vi "ReadCICDPathConfig.vi"(8 "error in (no error)":errorcluster, 11 "Workspace Path":path=path "E:/sw-deps-monitor") -> (0 "error out":errorcluster, 3 "CICD Path Config Out":T1)   [LabVIEW 2023, in "CheckModifiedVIs.lvlib"]
uses:
  CheckModifiedVIs/CheckModifiedVIs.lvlib
  Typedefs/CICDPathConfigs.ctl
  <vilib>/Utility/config.llb/NI_LVConfig.lvlib
  Reusables.lvlib
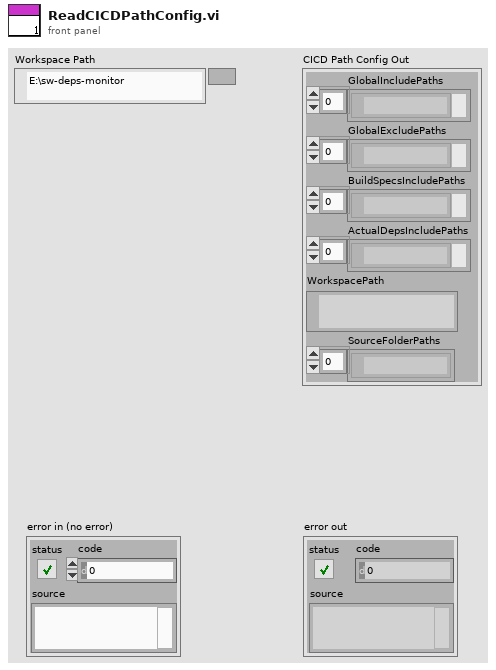
[diagram p1: front panel]
types:
  T1 = typedef "Reusables.lvlib/CICDPathConfigs.ctl" = cluster{"GlobalIncludePaths":path[], "GlobalExcludePaths":path[], "BuildSpecsIncludePaths":path[], "ActualDepsIncludePaths":path[], "WorkspacePath":path, "SourceFolderPaths":path[]}
  T2 = typedef "NI_LVConfig.lvlib/Config Data RefNum.ctl" = refnum<k1>
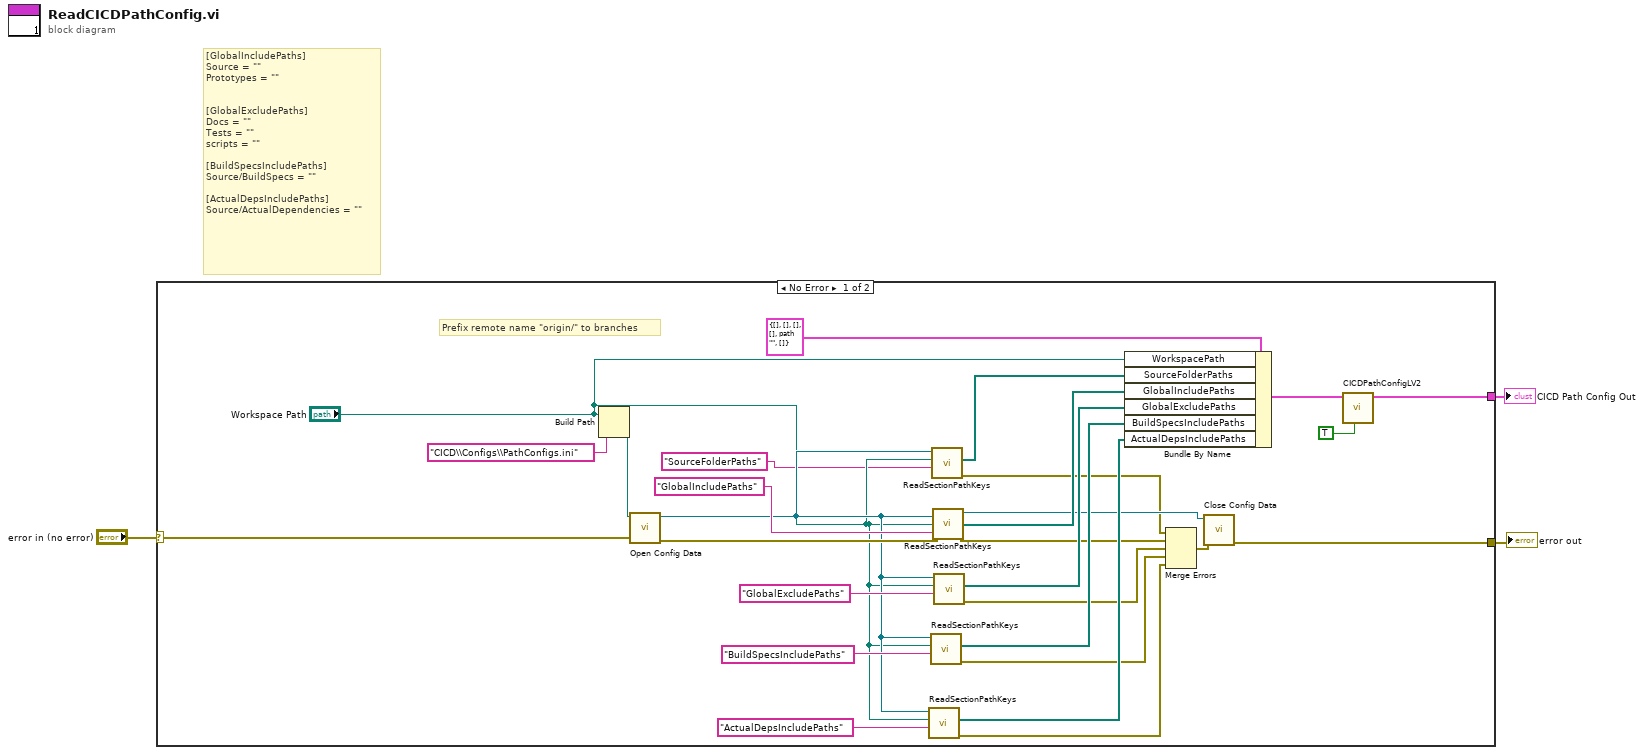
[diagram p0: block diagram]
diagram:
  # "[GlobalIncludePaths]\nSource = \"\"\nPrototypes = \"\"\n\n\n[GlobalExcludePaths]\nDocs = \"\"\nTests = \"\"\nscripts = \"\"\n\n[BuildSpecsIncludePaths]\nSource/BuildSpecs = \"\"\n\n[ActualDepsIncludePaths]\nSource/ActualDependencies = \"\""
  n1 = case shown="No Error" "error in (no error)" {
    selector: "error in (no error)" -> [w31 w32]
    tunnel: [w12 w32] -> w2
    tunnel: [w9 _] -> w1
    frame No Error {
      # "Prefix remote name \"origin/\" to branches"
      n2 = Build Path(base path="Workspace Path", name or relative path="CICD\\Configs\\PathConfigs.ini" ("CICD Path Config Rel")) -> (appended path=w30:path)
      n3 = call <vilib>:"Open Config Data.vi"("error in (no error)"=w31, "configuration file path"=w30) -> ("error out"=w28:errorcluster, "refnum"=w8:T2)  [unwired: 7 in, 1 out]
      n4 = call "ReadSectionPathKeys.vi"("section"="ActualDepsIncludePaths", "Workspace Path"="Workspace Path", "Refnum in"=w8) -> ("error out"=w15:errorcluster, "Paths"=w19:path[])  [unwired: 6 in, 1 out]
      n5 = call "ReadSectionPathKeys.vi"("section"="BuildSpecsIncludePaths", "Workspace Path"="Workspace Path", "Refnum in"=w8) -> ("error out"=w16:errorcluster, "Paths"=w20:path[])  [unwired: 6 in, 1 out]
      n6 = call "ReadSectionPathKeys.vi"("section"="SourceFolderPaths", "Workspace Path"="Workspace Path", "Refnum in"=w8) -> ("error out"=w5:errorcluster, "Paths"=w4:path[])  [unwired: 6 in, 1 out]
      n7 = call "ReadSectionPathKeys.vi"("error in (no error)"=w28, "section"="GlobalIncludePaths", "Workspace Path"="Workspace Path", "Refnum in"=w8) -> ("error out"=w18:errorcluster, "Paths"=w22:path[], "refnum out"=w13:T2)  [unwired: 5 in]
      n8 = call "ReadSectionPathKeys.vi"("section"="GlobalExcludePaths", "Workspace Path"="Workspace Path", "Refnum in"=w8) -> ("error out"=w17:errorcluster, "Paths"=w21:path[])  [unwired: 6 in, 1 out]
      n9 = Bundle By Name(cluster=T1 {"GlobalIncludePaths"=[], "GlobalExcludePaths"=[], "BuildSpecsIncludePaths"=[], "ActualDepsIncludePaths"=[], "WorkspacePath"=path "", "SourceFolderPaths"=[]}, "WorkspacePath"="Workspace Path", "SourceFolderPaths"=w4, "GlobalIncludePaths"=w22, "GlobalExcludePaths"=w21, "BuildSpecsIncludePaths"=w20, "ActualDepsIncludePaths"=w19) -> (w10:T1)
      n10 = Merge Errors(w5, w18, w17, w16, w15) -> (w14:errorcluster)
      n11 = call <vilib>:"Close Config Data.vi"("error in (no error)"=w14, "refnum"=w13) -> ("error out"=w12:errorcluster)  [unwired: 8 in, 1 out]
      n12 = call "CICDPathConfigLV2.vi"("Set? (F)"=TRUE, "CICD Path Config In"=w10) -> ("CICD Path Config Out"=w9:T1)  [unwired: 9 in]
    }
    frame Error {
    }
  }
  "error out" <- w2
  "CICD Path Config Out" <- w1
